vi "Running average 1D.vi"(9 "Filter half  Width":i32=1, 11 "Unfiltered Data":dbl[](array[numeric])=[1.0, 3.0, 5.0, nan, 1.0]) -> (3 "Filtered data out":dbl[](array[numeric])=[1.0, 2.0, 3.0, 3.0, 3.0])   [LabVIEW 2009]
uses:
  <vilib>/ptbypt/NI_PtbyPt.lvlib
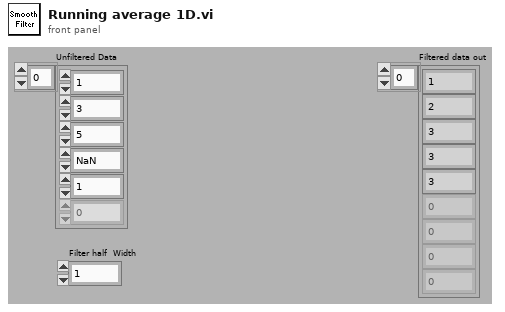
[diagram p1: front panel]
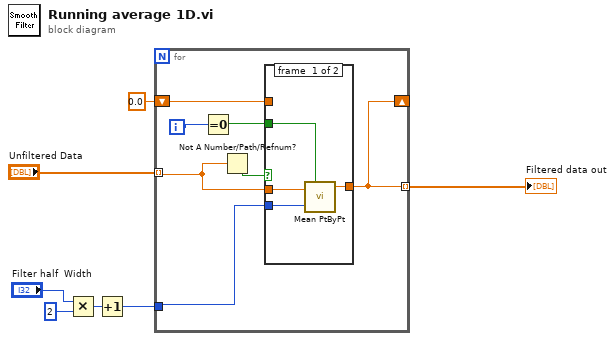
[diagram p0: block diagram]
diagram:
  n1 = Multiply(x="Filter half  Width", y=2) -> (x*y=w5:i32)
  n2 = Increment(x=w5) -> (x+1=w4:i32)
  n3 = for {
    tunnel: "Unfiltered Data" -> [w11] mode=indexing
    tunnel: w4 -> [w12]
    tunnel: [w8] -> w2 mode=indexing
    shift-right: [w8] -> _
    shift-left: 0.0 ("mean") -> [w9]
    i -> [w13]
    n4 = Equal To 0?(x=w13) -> (x = 0?=w14:bool)
    n5 = Not A Number/Path/Refnum?(number/path/refnum=w11) -> (NaN/Path/Refnum?=w10:bool)
    n6 = case shown="False" w10 {
      tunnel: w14 -> [w18 _]
      tunnel: w11 -> [w17 _]
      tunnel: w12 -> [w16 _]
      tunnel: [w15 w19] -> w8
      tunnel: w9 -> [_ w19]
      frame #0 {
        n7 = call <vilib>:"Mean PtByPt.vi"("x"=w17, "sample length"=w16, "initialize"=w18) -> ("mean"=w15:dbl)  [unwired: 2 out]
      }
      frame #1 {
      }
    }
  }
  "Filtered data out" <- w2
